vi "From BananaLeaf.Assert.vi"(11 "Leaf.Properties.Assert":refnum<class "Leaf.Properties.Assert.lvclass">) -> (2 "Properties.Assert":refnum<class "Properties.Assert.lvclass">)   [LabVIEW 2021, in "Banana.Caraya.lvlib" / "Leaf.Properties.Assert.lvclass"]
uses:
  Leaf.Properties.Assert.lvclass
  C:/Repositories/LVOS/Bananas/lv-src/Banana.Caraya/Leaf.Properties/Leaf.Properties.lvclass
  <vilib>/addons/_JKI Toolkits/Caraya/classes/Properties.Assert/Properties.Assert.lvclass
  Leaf.Properties/Leaf.Properties.lvclass/Leaf.Properties.ctl
  Leaf.Properties.Assert.lvclass/Leaf.Properties.Assert.ctl
  Leaf.Properties/Leaf.Properties.lvclass
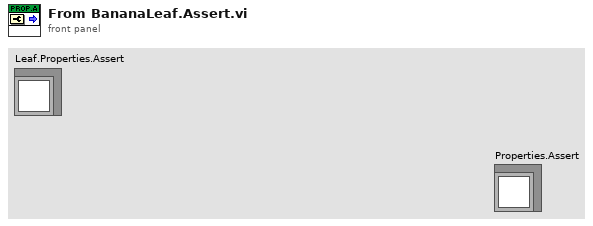
[diagram p1: front panel]
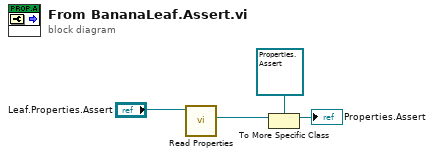
[diagram p0: block diagram]
diagram:
  n1 = call "Read Properties.vi"("Leaf.Properties in"="Leaf.Properties.Assert") -> ("Properties"=w3:refnum<class "Properties.lvclass">)  [unwired: 9 in, 1 out]
  n2 = To More Specific Class(target class=refnum<class "Properties.Assert.lvclass"> refnum ("Properties.Assert"), reference=w3) -> (specific class reference=→"Properties.Assert":refnum<class "Properties.Assert.lvclass">)  [unwired: 1 in, 1 out]
